vi "opCRD Server (9636-original).vi"   [LabVIEW 2013]
uses:
  CRD/tCRD.lvclass
  Reusable/Instrument/state.ctl
  Devices/Airmar/Data/Airmar Data.lvclass
  Devices/Airmar/Airmar WS.lvclass
  Reusable/Session APIs/File Access/Config Data/Config Session.ctl
  Reusable/Session APIs/File Access/Config Data/Config Data.lvclass
  Devices/Nephelometer/Nephelometer.lvclass
  Reusable/File IO/Class/File Observer.lvclass
  <vilib>/Platform/TimedLoop/XDataNode/timing_clust.ctl
  <vilib>/Platform/TimedLoop/XDataNode/nitl_modes.ctl
  <vilib>/Platform/TimedLoop/XDataNode/wakeup.ctl
  Reusable/CRDS/Main/CRDS.lvclass/CRDS.ctl
  Reusable/File IO/Class/File Observer.lvclass/File Observer.ctl
  Devices/Configurable Device/Configurable Device.lvclass/Configurable Device.ctl
  Devices/Airmar/Airmar WS.lvclass/Airmar WS.ctl
  Devices/Nephelometer/Nephelometer.lvclass/Nephelometer.ctl
  Devices/Configurable Device/Write Handle.vi
  Reusable/File IO/Class/Accessors/Write Top Data Path.vi
  Reusable/File IO/Class/Accessors/Write File Prefix.vi
  Reusable/File IO/Class/Accessors/Write File Ext.vi
  Reusable/File IO/Class/Accessors/Write File Header.vi
  Reusable/File IO/Class/Accessors/Write Max Size.vi
  Reusable/CRDS/Main/Read CRD RD Data Obs.vi
  Reusable/CRDS/Main/Write CRD RD Data Obs.vi
  <vilib>/nisyscfg/Close (System).vi
  Devices/Nephelometer/Unpolled Commands/Start_Stop Polling Mode.vi
  Devices/Nephelometer/Read Commands/Get Scatter Data.vi
  Devices/Nephelometer/Read Commands/Get Auxilary Data.vi
  <vilib>/Platform/TimedLoop/XDataNode/XDataNode.xnode
  Reusable/Instrument/Instrument.lvclass
  Reusable/Session APIs/Serial/Serial Session.lvclass
  <userlib>/_Session Fwk/Session - Root.lvclass
  <vilib>/Platform/TimedLoop/XDataNode/XDNodeRunTimeDep.lvlib
  <vilib>/nisyscfg/nisyscfg.lvlib
types:
  T1 = typedef "Config Data.lvclass/Config Session.ctl" = refnum<data-value>
  T2 = typedef "Instrument.lvclass/state.ctl" = enum8{"Configure", "Acquire", "Wait", "Quit", "Handle Error", "NOOP"}
  T3 = typedef "Session - Root.lvclass/Session Handle.ctl" = refnum<data-value>
  T4 = typedef "XDNodeRunTimeDep.lvlib/timing_clust.ctl" = cluster{"Expected End [f-1]":u64, "Actual End [f-1]":u64, "Finished Late? [f-1]":bool, "Expected End [i-1]":u64, "Actual End [i-1]":u64, "Finished Late? [i-1]":bool, "Expected Start [i]":u64, "Actual Start [i]":u64, "Expected Start [f]":u64, "Actual Start [f]":u64, "Source Name":string, "Structure Name":string, "Period":i64, "Deadline":i64, "Offset":i64, "Start":i64, "Priority":i32, "Timeout":i32, "Mode":T5, "Wakeup Reason":T6, "Error":errorcluster, "Source Type":string, "Secondary Source Type":string, "Global End Time":u64, "Global Start Time":u64, "Frame Duration":u64, "Iteration Duration":u64, "Assigned CPU":i32, "I/O Scan Engine Mode":u32}
  T5 = typedef "XDNodeRunTimeDep.lvlib/nitl_modes.ctl" = enum32{"No Change", "Process missed periods, maintain original phase", "Discard missed periods, maintain original phase", "Process missed periods, ignore original phase", "Discard missed periods, ignore original phase"}
  T6 = typedef "XDNodeRunTimeDep.lvlib/wakeup.ctl" = enum32{"Normal", "Aborted", "Asynchronous wakeup", "Timing source error", "Timed loop error", "Timeout"}
  T7 = typedef "Serial Session.lvclass/Session Handle.ctl" = refnum<data-value>
  T8 = cluster{"Mode":enum16{"Normal", "Zero", "Blank"}, "Scatter Mode":enum16{"Total Scatter", "Back Scatter"}, "Time in Mode":i32, "Cblue":dbl, "Cgreen":dbl, "Cred":dbl, "Cback,blue":dbl, "Cback,green":dbl, "Cback,red":dbl}
  T9 = cluster{"Sensitivity":dbl, "Pressure":dbl, "Tsample":dbl, "Tinlet":dbl, "RH":dbl, "Vlamp":dbl, "Ilamp":dbl}
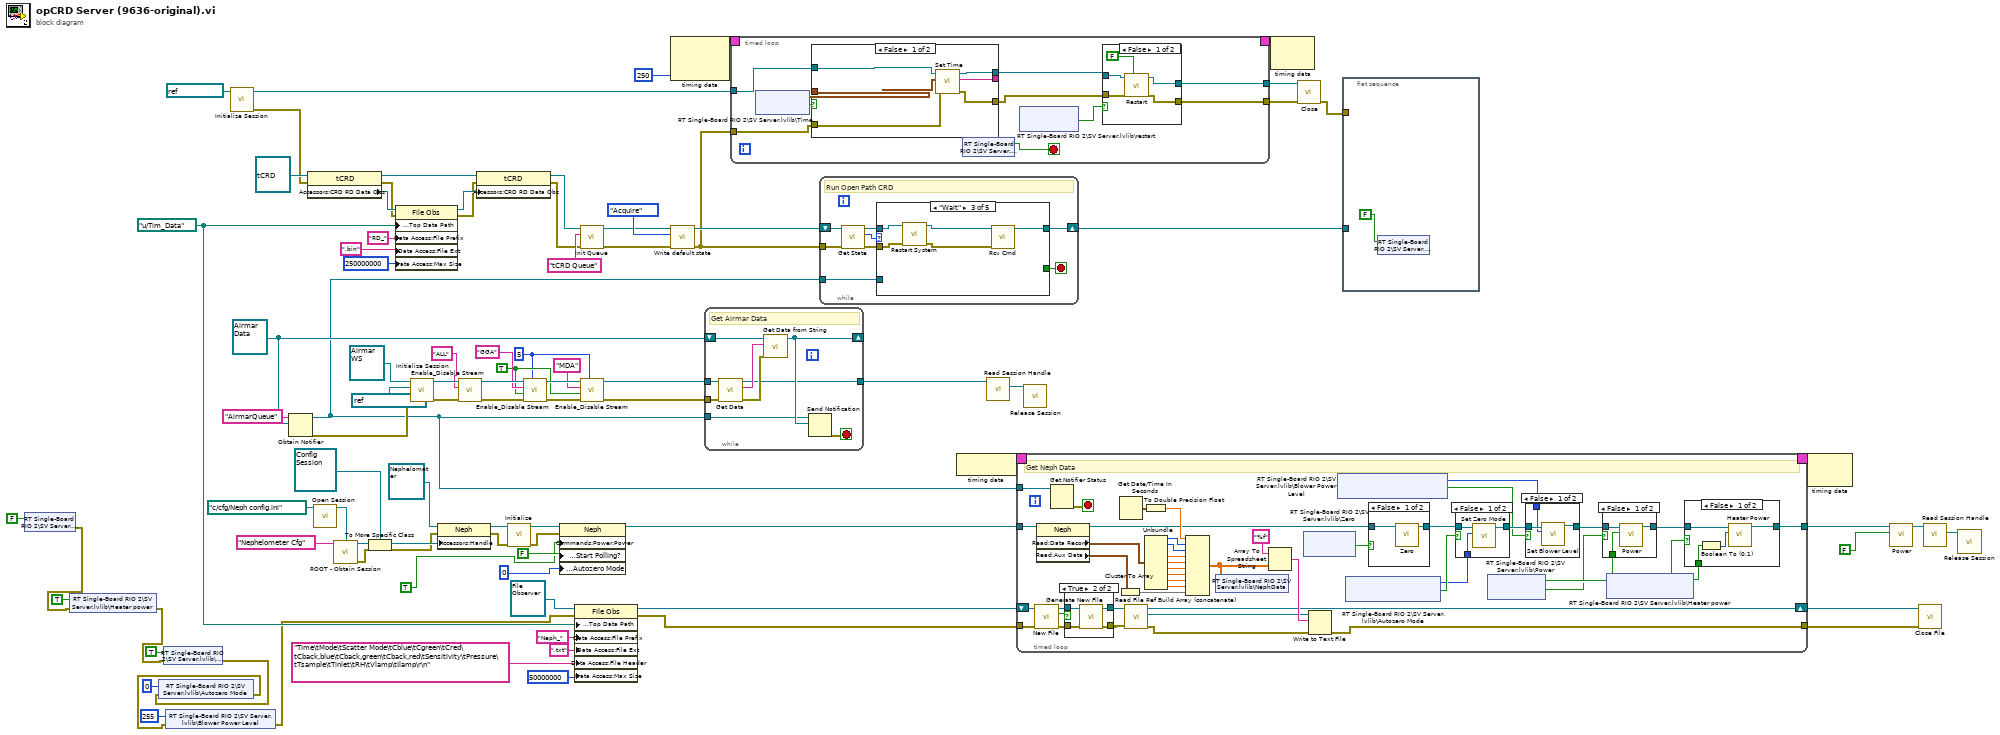
[diagram p0: block diagram]
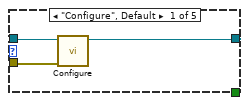
[diagram p10: hidden frame]
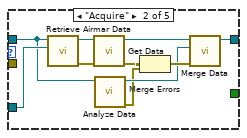
[diagram p11: hidden frame]
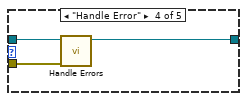
[diagram p12: hidden frame]
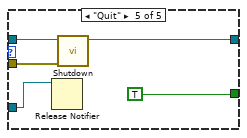
[diagram p13: hidden frame]
diagram:
  w35 = path "u:/Tim_Data" ("RD Data Path")
  w73 = i16 5 ("time")
  w74 = TRUE ("Enable?")
  w86 = refnum<class "Airmar Data.lvclass"> refnum ("Airmar Data")
  n1 = shared-variable "RT Single-Board RIO 2\\SV Server.lvlib\\Stop"(FALSE ("Stop")) -> (error out=w7:errorcluster)  [unwired: 1 in]
  n2 = shared-variable "RT Single-Board RIO 2\\SV Server.lvlib\\Heater power"(TRUE ("Heater power"), error in=w7) -> (error out=w20:errorcluster)
  n3 = shared-variable "RT Single-Board RIO 2\\SV Server.lvlib\\Power"(TRUE ("Blower Pwr"), error in=w20) -> (error out=w23:errorcluster)
  n4 = shared-variable "RT Single-Board RIO 2\\SV Server.lvlib\\Autozero Mode"(u8 0 ("Autozero Mode"), error in=w23) -> (error out=w22:errorcluster)
  n5 = shared-variable "RT Single-Board RIO 2\\SV Server.lvlib\\Blower Power Level"(u8 255 ("Blower Power Level"), error in=w22) -> (error out=w21:errorcluster)
  n6 = call <vilib>:"Initialize Session.vi"("target (localhost)"=refnum<k21> "localhost") -> ("error out"=w4:errorcluster, "session out"=w5:refnum<k21>)  [unwired: 9 in]
  n7 = Obtain Notifier(name (unnamed)="AirmarQueue", notification data type=w86) -> (notifier out=w55:refnum<notifier>, error out=w84:errorcluster)  [unwired: 2 in, 1 out]
  n8 = property class="tCRD"(reference=refnum<class "tCRD.lvclass"> refnum ("tCRD"), error in=w4) -> (reference out=w65:refnum<class "tCRD.lvclass">, error out=w62:errorcluster, "Accessors:CRD RD Data Obs"=w64:refnum<class "File Observer.lvclass">)
  n9 = call "Open Session.vi"("Path"=path "c:/cfg/Neph config.ini") -> ("Config Data"=w54:refnum<class "Config Data.lvclass">)  [unwired: 9 in, 1 out]
  n10 = call <userlib>:"ROOT - Obtain Session.vi"("Session Name ()"="Nephelometer Cfg", "OBJ - Session"=w54) -> ("Session Handle"=w51:T3, "error out"=w50:errorcluster)  [unwired: 11 in, 1 out]
  n11 = To More Specific Class(target class=T1 refnum ("Session Handle"), reference=w51, error in=w50) -> (specific class reference=w48:T1, error out=w47:errorcluster)
  n12 = property class="File Obs"(reference=w64, error in=w62, "Data Access:Top Data Path"=w35, "Data Access:File Prefix"="RD_" ("File Prefix"), "Data Access:File Ext"=".bin" ("File Prefix"), "Data Access:Max Size"=i64 250000000 ("Max Size")) -> (reference out=w63:refnum<class "File Observer.lvclass">, error out=w61:errorcluster)
  n13 = call <vilib>:"Initialize Session.vi"("error in"=w84, "VISA Resource"=refnum<visa-resource-name> "ASRL3::INSTR", "Airmar WS in"=refnum<class "Airmar WS.lvclass"> refnum) -> ("error out"=w67:errorcluster, "Airmar WS out"=w81:refnum<class "Airmar WS.lvclass">)  [unwired: 7 in]
  n14 = property class="Neph"(reference=refnum<class "Nephelometer.lvclass"> refnum ("Neph"), error in=w47, "Accessors:Handle"=w48) -> (reference out=w46:refnum<class "Nephelometer.lvclass">, error out=w45:errorcluster)
  n15 = call "Enable_Disable Stream.vi"("error in (no error)"=w67, "String"="ALL", "Airmar WS in"=w81) -> ("error out"=w68:errorcluster, "Airmar WS out"=w79:refnum<class "Airmar WS.lvclass">)  [unwired: 7 in]
  n16 = property class="tCRD"(reference=w65, error in=w61, "Accessors:CRD RD Data Obs"=w63) -> (reference out=w58:refnum<class "tCRD.lvclass">, error out=w57:errorcluster)
  n17 = call "Initialize.vi"("error in"=w45, "Neph In"=w46) -> ("error out"=w38:errorcluster, "Neph Out"=w40:refnum<class "Nephelometer.lvclass">)  [unwired: 8 in]
  n18 = call "Enable_Disable Stream.vi"("time"=w73, "error in (no error)"=w68, "Enable?"=w74, "String"="GGA", "Airmar WS in"=w79) -> ("error out"=w76:errorcluster, "Airmar WS out"=w77:refnum<class "Airmar WS.lvclass">)  [unwired: 5 in]
  n19 = property class="Neph"(reference=w40, error in=w38, "Commands:Power:Power"=TRUE ("Power?"), "Commands:Polling:Start Polling?"=FALSE ("Start Polling?"), "Commands:Autozero Mode"=u8 0 ("Zero Mode")) -> (reference out=w37:refnum<class "Nephelometer.lvclass">)  [unwired: 1 out]
  n20 = property class="File Obs"(reference=refnum<class "File Observer.lvclass"> refnum ("File Obs"), error in=w21, "Data Access:Top Data Path"=w35, "Data Access:File Prefix"="Neph_" ("File Prefix"), "Data Access:File Ext"=".txt" ("File Ext"), "Data Access:File Header"="Time\tMode\tScatter Mode\tCblue\tCgreen\tCred\tCback,blue\tCback,green\tCback,red\tSensitivity\tPressure\tTsample\tTinlet\tRH\tVlamp\tIlamp\r\n" ("File Header"), "Data Access:Max Size"=i64 50000000 ("Max Size")) -> (reference out=w31:refnum<class "File Observer.lvclass">, error out=w30:errorcluster)
  n21 = call "Init Queue.vi"("error in"=w57, "queue_name"="tCRD Queue", "Instrument in"=w58) -> ("error out"=w87:errorcluster, "Instrument out"=w88:refnum<class "tCRD.lvclass">)  [unwired: 7 in]
  n22 = call "Enable_Disable Stream.vi"("time"=w73, "error in (no error)"=w76, "Enable?"=w74, "String"="MDA", "Airmar WS in"=w77) -> ("error out"=w71:errorcluster, "Airmar WS out"=w72:refnum<class "Airmar WS.lvclass">)  [unwired: 5 in]
  n23 = node-c288(i64 250 ("Period")) -> (w12:T4)  [unwired: 1 in]
  n24 = call "Write default state.vi"("error in (no error)"=w87, "instr state"=state."Acquire", "Instrument in"=w88) -> ("error out"=w9:errorcluster, "Instrument out"=w89:refnum<class "tCRD.lvclass">)  [unwired: 7 in]
  n25 = while {
    tunnel: w72 -> [w100]
    shift-right: [w96] -> _
    shift-left: w86 -> [w98]
    tunnel: w55 -> [w95]
    tunnel: [w93] -> w70
    tunnel: w71 -> [w92]
    stop <- w94 stop-if-true
    # "Get Airmar Data"
    n26 = call "Get Data.vi"("error in"=w92, "Airmar WS in"=w100) -> ("error out"=w97:errorcluster, "Data"=w99:string, "Airmar WS out"=w93:refnum<class "Airmar WS.lvclass">)  [unwired: 7 in]
    n27 = call "Get Data from String.vi"("error in (no error)"=w97, "DataIn"=w99, "Airmar Data in"=w98) -> ("Airmar Data out"=w96:refnum<class "Airmar Data.lvclass">)  [unwired: 7 in, 1 out]
    n28 = Send Notification(notification=w96, notifier=w95) -> (error out=w94:errorcluster)  [unwired: 1 in, 1 out]
  }
  n29 = timed-loop {
    timing: w12 -> [_]
    timing-out: [_] -> w11
    tunnel: w9 -> [w106]
    tunnel: w5 -> [w107]
    tunnel: [w104] -> w3
    tunnel: [w102] -> w1
    stop <- w108 stop-if-true
    n30 = shared-variable "RT Single-Board RIO 2\\SV Server.lvlib\\Time"() -> (w109:timestamp, w110:bool)  [unwired: 2 in, 1 out]
    n31 = case shown="False" w110 {
      tunnel: w109 -> [w123 _]
      tunnel: [w122 _] -> _
      tunnel: w107 -> [w121 w125]
      tunnel: [w120 w125] -> w105
      tunnel: w106 -> [w119 w124]
      tunnel: [w118 w124] -> w103
      frame False {
        n32 = call <vilib>:"Set Time.vi"("error in (no error)"=w119, "time"=w123, "session in (localhost)"=w121) -> ("error out"=w118:errorcluster, "detailed result"=w122:string, "session out"=w120:refnum<k21>)  [unwired: 5 in, 1 out]
      }
      frame True {
      }
    }
    n33 = shared-variable "RT Single-Board RIO 2\\SV Server.lvlib\\Stop"() -> (w108:bool)  [unwired: 1 in, 1 out]
    n34 = shared-variable "RT Single-Board RIO 2\\SV Server.lvlib\\restart"() -> (w101:bool)  [unwired: 2 in, 2 out]
    n35 = case shown="False" w101 {
      tunnel: w105 -> [w115 w117]
      tunnel: [w114 w117] -> w104
      tunnel: w103 -> [w112 w116]
      tunnel: [w111 w116] -> w102
      frame False {
        n36 = call <vilib>:"Restart.vi"("wait until complete (T)"=FALSE, "error in (no error)"=w112, "session in"=w115) -> ("error out"=w111:errorcluster, "session out"=w114:refnum<k21>)  [unwired: 6 in, 1 out]
      }
      frame True {
      }
    }
  }
  n37 = while "Acquisition" {
    tunnel: w9 -> [w135]
    shift-right: [w129] -> w13
    shift-left: w89 -> [w133]
    tunnel: w55 -> [w128]
    stop <- w130 stop-if-true
    # "Run Open Path CRD"
    n38 = call "Get State.vi"("error in"=w135, "Instrument in"=w133) -> ("error out"=w131:errorcluster, "default state"=w134:T2, "Instrument out"=w132:refnum<class "tCRD.lvclass">)  [unwired: 7 in]
    n39 = case shown="\"Wait\"" w134 {
      tunnel: w132 -> [w138 w140 w152 w156 w160]
      tunnel: w131 -> [w137 _ w151 w155 w159]
      tunnel: [_ _ _ _ TRUE] -> w130
      tunnel: [w136 w148 w153 w154 w158] -> w129
      tunnel: w128 -> [_ w142 _ _ w157]
      frame "Configure", Default {
        n40 = call-dynamic "Configure.vi"("error in"=w137, "tCRD in"=w138) -> ("tCRD out"=w136:refnum<class "tCRD.lvclass">)  [unwired: 8 in, 1 out]
      }
      frame "Acquire" {
        n41 = call "Retrieve Airmar Data.vi"("AirMar Data"=w142, "tCRD in"=w140) -> ("error out"=w139:errorcluster, "tCRD out"=w141:refnum<class "tCRD.lvclass">)  [unwired: 8 in]
        n42 = call-dynamic "Get Data.vi"("error in"=w139, "tCRD in"=w141) -> ("error out"=w144:errorcluster, "tCRD out"=w147:refnum<class "tCRD.lvclass">)  [unwired: 8 in]
        n43 = call-dynamic "Analyze Data.vi"("CRDS in"=w140) -> ("error out"=w143:errorcluster, "CRDS out"=w145:refnum<class "tCRD.lvclass">)  [unwired: 9 in]
        n44 = Merge Errors(w144, w143) -> (w146:errorcluster)
        n45 = call-dynamic "Merge Data.vi"("error in"=w146, "Analyzed"=w145, "Acquired"=w147) -> ("tCRD out"=w148:refnum<class "tCRD.lvclass">)  [unwired: 7 in, 1 out]
      }
      frame "Wait" {
        n46 = call "Restart System.vi"("error in (no error)"=w151, "tCRD in"=w152) -> ("error out"=w149:errorcluster, "tCRD out"=w150:refnum<class "tCRD.lvclass">)  [unwired: 8 in]
        n47 = call-dynamic "Rcv Cmd.vi"("error in"=w149, "tCRD in"=w150) -> ("tCRD out"=w153:refnum<class "tCRD.lvclass">)  [unwired: 8 in, 1 out]
      }
      frame "Handle Error" {
        n48 = call-dynamic "Handle Errors.vi"("error in"=w155, "tCRD in"=w156) -> ("tCRD out"=w154:refnum<class "tCRD.lvclass">)  [unwired: 7 in, 2 out]
      }
      frame "Quit" {
        n49 = Release Notifier(notifier=w157) -> ()  [unwired: 2 in, 3 out]
        n50 = call-dynamic "Shutdown.vi"("error in"=w159, "tCRD in"=w160) -> ("tCRD out"=w158:refnum<class "tCRD.lvclass">)  [unwired: 8 in, 1 out]
      }
    }
  }
  n51 = node-c288() -> (w42:T4)
  n52 = call "Read Session Handle.vi"("Airmar WS in"=w70) -> ("Session Handle"=w69:T7)  [unwired: 8 in, 2 out]
  n53 = timed-loop {
    tunnel: w37 -> [w206]
    tunnel: w55 -> [w205]
    tunnel: [w164] -> w18
    timing: w42 -> [_]
    timing-out: [_] -> w41
    tunnel: w30 -> [w202]
    tunnel: [w178] -> w28
    shift-right: [w179] -> w29
    shift-left: w31 -> [w203]
    stop <- w204 stop-if-true
    # "Get Neph Data"
    n54 = call-dynamic "New File.vi"("error in"=w202, "File Observer in"=w203) -> ("error out"=w199:errorcluster, "Exceeded"=w201:bool, "File Observer out"=w200:refnum<class "File Observer.lvclass">)  [unwired: 7 in]
    n55 = property class="Neph"(reference=w206) -> (reference out=w176:refnum<class "Nephelometer.lvclass">, "Read:Data Record"=w198:T8, "Read:Aux Data"=w190:T9)  [unwired: 1 in, 1 out]
    n56 = Get Notifier Status(notifier=w205) -> (error out=w204:errorcluster)  [unwired: 1 in, 4 out]
    n57 = case shown="True" w201 {
      tunnel: w200 -> [w228 w232]
      tunnel: w199 -> [w227 w231]
      tunnel: [w228 w230] -> w185
      tunnel: [w227 w229] -> w184
      frame False {
      }
      frame True {
        n58 = call-dynamic "Generate New File.vi"("error in"=w231, "File Obs in"=w232) -> ("error out"=w229:errorcluster, "File Obs out"=w230:refnum<class "File Observer.lvclass">)  [unwired: 7 in, 1 out]
      }
    }
    n59 = Cluster To Array(cluster=w190) -> (array=w186:dbl[])
    n60 = Get Date/Time In Seconds() -> (seconds since 1Jan1904=w191:timestamp)
    n61 = call "Read File Ref.vi"("error in"=w184, "File Observer in"=w185) -> ("error out"=w180:errorcluster, "File Ref"=w181:refnum<file>, "File Observer out"=w179:refnum<class "File Observer.lvclass">)  [unwired: 7 in]
    n62 = To Double Precision Float(number=w191) -> (double precision float=w187:dbl)
    n63 = Unbundle(w198) -> ("Mode"=w188:enum16{"Normal", "Zero", "Blank"}, "Scatter Mode"=w189:enum16{"Total Scatter", "Back Scatter"}, "Cblue"=w197:dbl, "Cgreen"=w196:dbl, "Cred"=w195:dbl, "Cback,blue"=w194:dbl, "Cback,green"=w193:dbl, "Cback,red"=w192:dbl)  [unwired: 1 out]
    n64 = Build Array (concatenate)(w187, w188, w189, w197, w196, w195, w194, w193, w192, w186) -> (w177:dbl[])
    n65 = shared-variable "RT Single-Board RIO 2\\SV Server.lvlib\\NephData"(w177) -> ()  [unwired: 1 in, 1 out]
    n66 = Array To Spreadsheet String(array=w177, 3:"%f" ("format string")) -> (spreadsheet string=w182:string)  [unwired: 1 in]
    n67 = shared-variable "RT Single-Board RIO 2\\SV Server.lvlib\\Zero"() -> (w175:bool)  [unwired: 2 in, 2 out]
    n68 = Write to Text File(file (use dialog)=w181, text=w182, error in=w180) -> (error out=w178:errorcluster)  [unwired: 1 in, 2 out]
    n69 = shared-variable "RT Single-Board RIO 2\\SV Server.lvlib\\Blower Power Level"() -> (w169:u8, w170:bool)  [unwired: 2 in, 1 out]
    n70 = shared-variable "RT Single-Board RIO 2\\SV Server.lvlib\\Autozero Mode"() -> (w172:u8, w174:bool)  [unwired: 2 in, 1 out]
    n71 = case shown="False" w175 {
      tunnel: w176 -> [w225 w226]
      tunnel: [w224 w226] -> w173
      frame False {
        n72 = call "Zero.vi"("Neph in"=w225) -> ("Neph out"=w224:refnum<class "Nephelometer.lvclass">)  [unwired: 9 in, 1 out]
      }
      frame True {
      }
    }
    n73 = case shown="False" w174 {
      tunnel: w173 -> [w222 w223]
      tunnel: [w221 w223] -> w171
      tunnel: w172 -> [w220 _]
      frame False {
        n74 = call "Set Zero Mode.vi"("Mode"=w220, "Neph in"=w222) -> ("Neph out"=w221:refnum<class "Nephelometer.lvclass">)  [unwired: 8 in, 1 out]
      }
      frame True {
      }
    }
    n75 = shared-variable "RT Single-Board RIO 2\\SV Server.lvlib\\Power"() -> (w167:bool, w166:bool)  [unwired: 2 in, 1 out]
    n76 = case shown="False" w170 {
      tunnel: w171 -> [w218 w219]
      tunnel: [w217 w219] -> w168
      tunnel: w169 -> [w216 _]
      frame False {
        n77 = call "Set Blower Level.vi"("Level"=w216, "Neph in"=w218) -> ("Neph out"=w217:refnum<class "Nephelometer.lvclass">)  [unwired: 8 in, 1 out]
      }
      frame True {
      }
    }
    n78 = case shown="False" w166 {
      tunnel: w168 -> [w214 w215]
      tunnel: [w213 w215] -> w165
      tunnel: w167 -> [w212 _]
      frame False {
        n79 = call "Power.vi"("Power?"=w212, "Neph in"=w214) -> ("Neph out"=w213:refnum<class "Nephelometer.lvclass">)  [unwired: 8 in, 1 out]
      }
      frame True {
      }
    }
    n80 = shared-variable "RT Single-Board RIO 2\\SV Server.lvlib\\Heater power"() -> (w162:bool, w163:bool)  [unwired: 2 in, 1 out]
    n81 = case shown="False" w163 {
      tunnel: w165 -> [w210 w211]
      tunnel: [w209 w211] -> w164
      tunnel: w162 -> [w208 _]
      frame False {
        n82 = Boolean To (0,1)(Boolean=w208) -> (0, 1=w207:i16)
        n83 = call "Heater Power.vi"("On/Off"=w207, "Neph in"=w210) -> ("Neph out"=w209:refnum<class "Nephelometer.lvclass">)  [unwired: 8 in, 1 out]
      }
      frame True {
      }
    }
  }
  n84 = call "Release Session.vi"("Session Handle"=w69) -> ()  [unwired: 14 in, 1 out]
  n85 = node-c288(w11) -> ()  [unwired: 1 out]
  n86 = call-poly <vilib>:"Close.vi"("error in (no error)"=w1, "session in"=w3) -> ("error out"=w2:errorcluster)  [unwired: 9 in]
  n87 = flat-sequence {
    tunnel: w13 -> [_]
    tunnel: w2 -> [_]
    frame #0 {
      n88 = shared-variable "RT Single-Board RIO 2\\SV Server.lvlib\\Stop"(FALSE ("Stop")) -> ()  [unwired: 1 in, 1 out]
    }
  }
  n89 = node-c288(w41) -> ()  [unwired: 1 out]
  n90 = call "Power.vi"("Power?"=FALSE, "Neph in"=w18) -> ("Neph out"=w17:refnum<class "Nephelometer.lvclass">)  [unwired: 8 in, 1 out]
  n91 = call-dynamic "Close File.vi"("error in"=w28, "File Obs in"=w29) -> ()  [unwired: 8 in, 2 out]
  n92 = call "Read Session Handle.vi"("Nephelometer in"=w17) -> ("Session Handle"=w43:T7)  [unwired: 8 in, 2 out]
  n93 = call "Release Session.vi"("Session Handle"=w43) -> ()  [unwired: 14 in, 1 out]
